vi "CMD StartDaq.vi"(8 "error in (no error)":errorcluster, 10 "vData":variant, 11 "DAQ in":refnum<class "DAQ.lvclass">) -> (0 "error out":errorcluster, 3 "DAQ out":refnum<class "DAQ.lvclass">)   [LabVIEW 2017, in "DAQ.lvclass"]
doc: "Developed by Kevin Thompson\nkevin@thompsonengineering.net\n\nCopyright 2018-2020\nThompson Engineering, LLC"
uses:
  DAQ.lvclass
  DataTypes/AsyncCmd_DAQ--enum.ctl
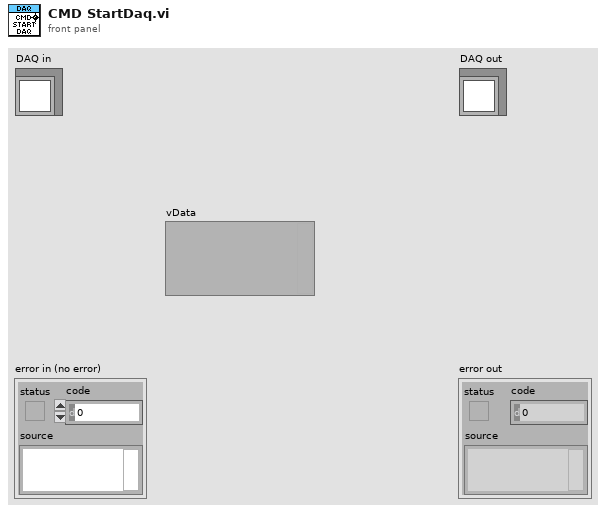
[diagram p1: front panel]
types:
  T1 = typedef "DAQ.lvclass/AsyncCmd_DAQ--enum.ctl" = enum16{"StartDAQ", "StopDAQ", "CfgDAQ"}
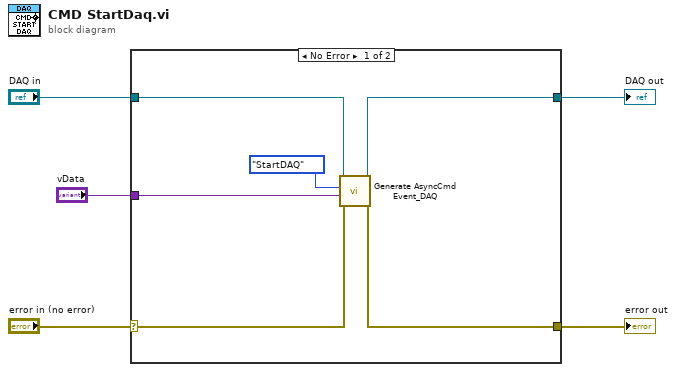
[diagram p0: block diagram]
diagram:
  n1 = case shown="No Error" "error in (no error)" {
    selector: "error in (no error)" -> [w11 w13]
    tunnel: [w10 w13] -> w4
    tunnel: [w8 w12] -> w2
    tunnel: "DAQ in" -> [w9 w12]
    tunnel: "vData" -> [w6 _]
    frame No Error {
      n2 = call "Generate AsyncCmd Event_DAQ.vi"("error in (no error)"=w11, "vData"=w6, "AsyncCmd"=AsyncCmd_DAQ--enum."StartDAQ" ("AsyncMsg"), "DAQ"=w9) -> ("error out"=w10:errorcluster, "DAQ out"=w8:refnum<class "DAQ.lvclass">)  [unwired: 6 in]
    }
    frame Error {
    }
  }
  "error out" <- w4
  "DAQ out" <- w2
